vi "addConvFeatureMap.vi"(0 "error in (no error)":errorcluster, 1 "stride":u32, 2 "ptr":i64, 3 "features":u32, 4 "kernelXY":u32, 5 "NOUTXY":u32) -> (6 "error out":errorcluster, 7 "ptr out":i64, 8 "layers":u32)   [LabVIEW 2016, in "CNet.lvlib"]
uses:
  CNet.lvlib
  Users/jg754/Documents/Visual Studio 2015/Projects/CLearn/x64/Debug/CLearn.dll
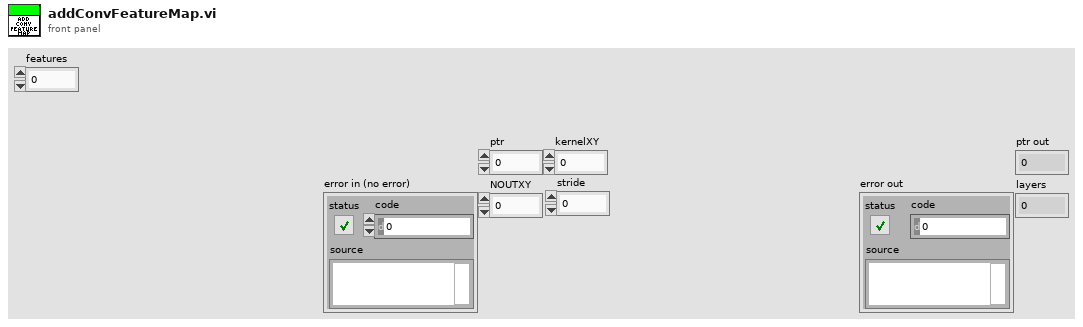
[diagram p1: front panel]
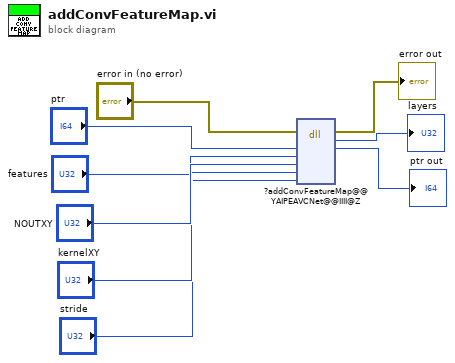
[diagram p0: block diagram]
diagram:
  n1 = dll-call lib="C:/Users/jg754/Documents/Visual Studio 2015/Projects/CLearn/x64/Debug/CLearn.dll" fn="?addConvFeatureMap@@YAIPEAVCNet@@IIII@Z"(error in="error in (no error)", "ptr"="ptr", "features"="features", "feature_NOUTXY"="NOUTXY", "feature_kernelXY"="kernelXY", "feature_stride"="stride") -> (error out=→"error out":errorcluster, "layers"=→"layers":u32, "ptr"=→"ptr out":i64)  [unwired: 6 in, 1 out]
